vi "Setup UI.vi"(8 "error in (no error)":errorcluster, 10 "Set UI to input?":bool, 11 "File IO in":refnum<class "File IO.lvclass">) -> (0 "error out":errorcluster, 3 "File IO out":refnum<class "File IO.lvclass">)   [LabVIEW 2017, in "File IO.lvclass"]
uses:
  File IO.lvclass
  File IO.lvclass/File IO.ctl
panel:
  in  "Light Source":string
  in  "Comments":string
  in  "File Path":path
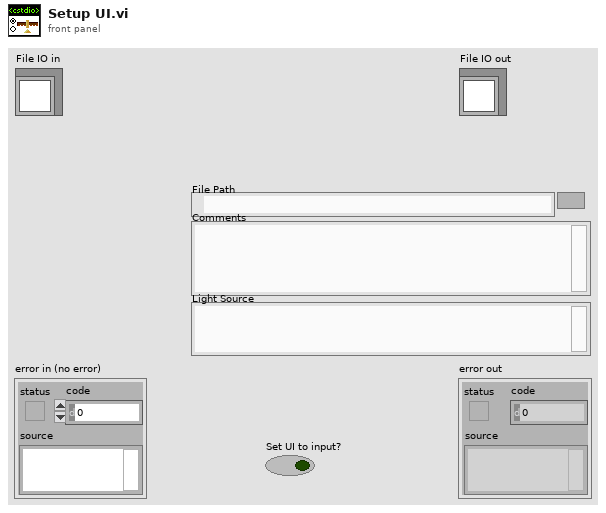
[diagram p1: front panel]
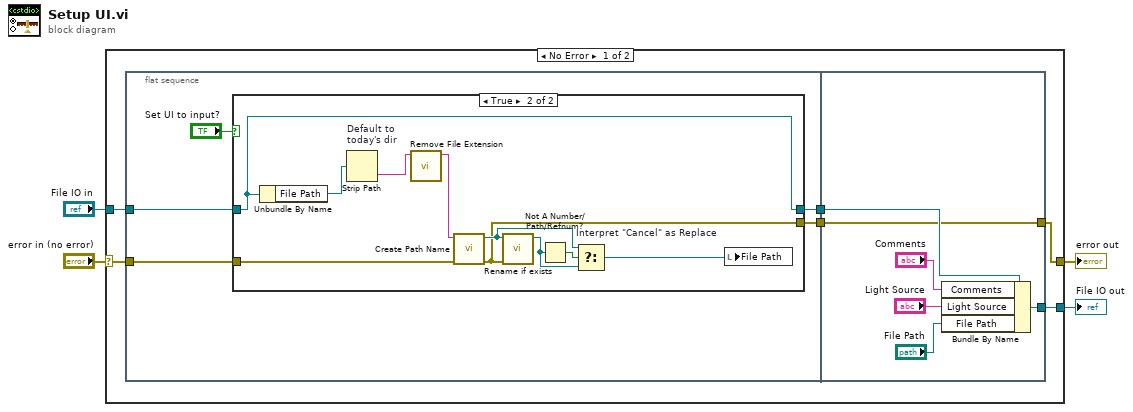
[diagram p0: block diagram]
diagram:
  n1 = case shown="No Error" "error in (no error)" {
    selector: "error in (no error)" -> [w7 w35]
    tunnel: [w5 w35] -> w3
    tunnel: [w9 w34] -> w1
    tunnel: "File IO in" -> [w10 w34]
    frame No Error {
      n2 = flat-sequence {
        tunnel: w10 -> [w14]
        tunnel: [w13] -> w8
        tunnel: w7 -> [w12]
        tunnel: [w11] -> w6
        tunnel: [w33] -> w9
        tunnel: w8 -> [w30]
        tunnel: w6 -> [w28]
        tunnel: [w28] -> w5
        frame #0 {
          n3 = case shown="True" "Set UI to input?" {
            tunnel: w14 -> [w16 w27]
            tunnel: [w16 w27] -> w13
            tunnel: w12 -> [w17 w25]
            tunnel: [w17 w18] -> w11
            frame False {
            }
            frame True {
              n4 = Unbundle By Name(w27) -> ("File Path"=w26:path)
              n5 = Strip Path "Default to\ntoday's dir"(path=w26) -> (name=w24:string)  [unwired: 1 out]
              n6 = call "Remove File Extension.vi"("filename"=w24) -> ("adjustedfilename"=w23:string)  [unwired: 6 out]
              n7 = call "Create Path Name.vi"("error in"=w25, "filename"=w23) -> ("error out"=w18:errorcluster, "path"=w20:path)  [unwired: 4 out]
              n8 = call "Rename if exists.vi"("error in"=w18, "File Path"=w20) -> ("New path"=w22:path)  [unwired: 1 in, 8 out]
              n9 = Not A Number/Path/Refnum?(number/path/refnum=w22) -> (NaN/Path/Refnum?=w21:bool)
              n10 = Select "Interpret \"Cancel\" as Replace"(t=w20, s=w21, f=w22) -> (s? t:f=w19:path)
              n11 = local write "File Path"(w19) -> ()
            }
          }
        }
        frame #1 {
          n12 = Bundle By Name(cluster=w30, "Comments"="Comments", "Light Source"="Light Source", "File Path"="File Path") -> (w33:refnum<class "File IO.lvclass">)
        }
      }
    }
    frame Error {
    }
  }
  "error out" <- w3
  "File IO out" <- w1
